vi "m1m3_getNextSample_ForceActuatorData.vi"(8 "error in (no error)":errorcluster, 11 "ForceActuatorData_Ctl":T1) -> (0 "error out":errorcluster, 2 "function return":i32, 3 "ForceActuatorData_Ctl out":T1)   [LabVIEW 2016, in "SALLV_m1m3.lvlib"]
doc: "int m1m3_shm_getNextSample_ForceActuatorDataLV(m1m3_ForceActuatorDataLV *ForceActuatorData_Ctl );"
uses:
  SALLV_m1m3.lvlib
  DataTypes/ForceActuatorData.ctl
  SALLV_m1m3.so
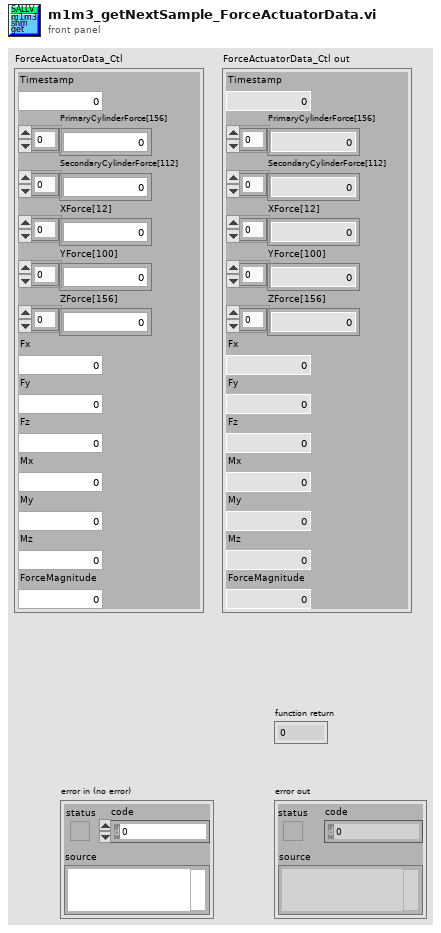
[diagram p1: front panel]
types:
  T1 = typedef "SALLV_m1m3.lvlib/ForceActuatorData.ctl" = cluster{"Timestamp":dbl, "PrimaryCylinderForce[156]":sgl[], "SecondaryCylinderForce[112]":sgl[], "XForce[12]":sgl[], "YForce[100]":sgl[], "ZForce[156]":sgl[], "Fx":sgl, "Fy":sgl, "Fz":sgl, "Mx":sgl, "My":sgl, "Mz":sgl, "ForceMagnitude":sgl}
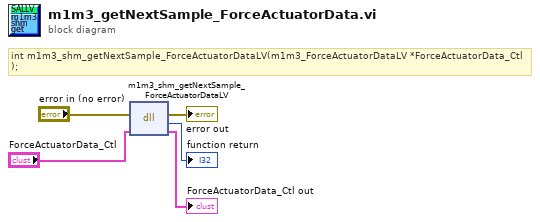
[diagram p0: block diagram]
diagram:
  # "int m1m3_shm_getNextSample_ForceActuatorDataLV(m1m3_ForceActuatorDataLV *ForceActuatorData_Ctl );"
  n1 = dll-call lib="opt/CODE/SALLV_m1m3/SALLV_m1m3.*" fn="m1m3_shm_getNextSample_ForceActuatorDataLV"(error in="error in (no error)", "ForceActuatorData_Ctl"="ForceActuatorData_Ctl") -> (error out=→"error out":errorcluster, →"function return":i32, "ForceActuatorData_Ctl"=→"ForceActuatorData_Ctl out":T1)  [unwired: 2 in, 1 out]
